vi "调试模式.vi"() -> ()   [LabVIEW 2018]
panel:
  out "开盖指令2":bool
  out "开盖指令1":bool
  out "压紧到位":bool
  out "锁定到位":bool
  out "开盖缓冲":bool
  out "开盖到位2":bool
  out "松开到位":bool
  out "开盖到位1":bool
  out "解锁到位":bool
  out "关盖缓冲":bool
  out "关盖到位2":bool
  out "关盖到位1":bool
  out "关盖指令2":bool
  out "关盖指令1":bool
  out "关盖换向阀":bool
  out "压紧换向阀":bool
  out "松开换向阀":bool
  out "开盖换向阀":bool
  in  "停止":bool
  in  "解锁":bool
  in  "锁定":bool
  in  "压紧":bool
  in  "关盖":bool
  in  "开盖":bool
  in  "松开":bool
  in  "井盖8":bool
  in  "井盖7":bool
  in  "井盖6":bool
  in  "井盖5":bool
  in  "井盖4":bool
  in  "井盖3":bool
  in  "井盖2":bool
  in  "井盖1":bool
  # "显示面板"
  # "操作面板"
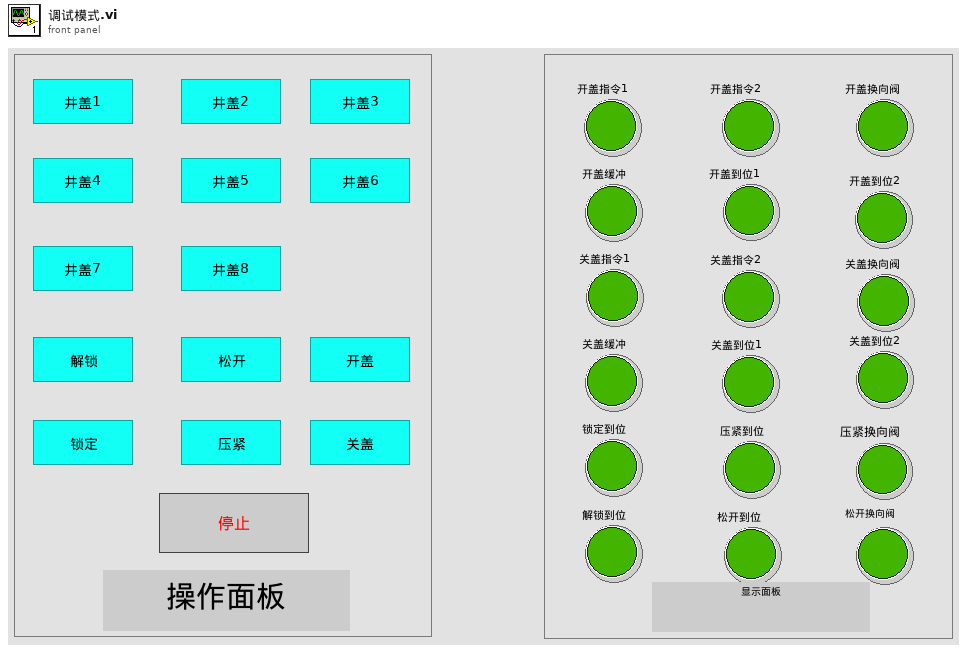
[diagram p1: front panel]
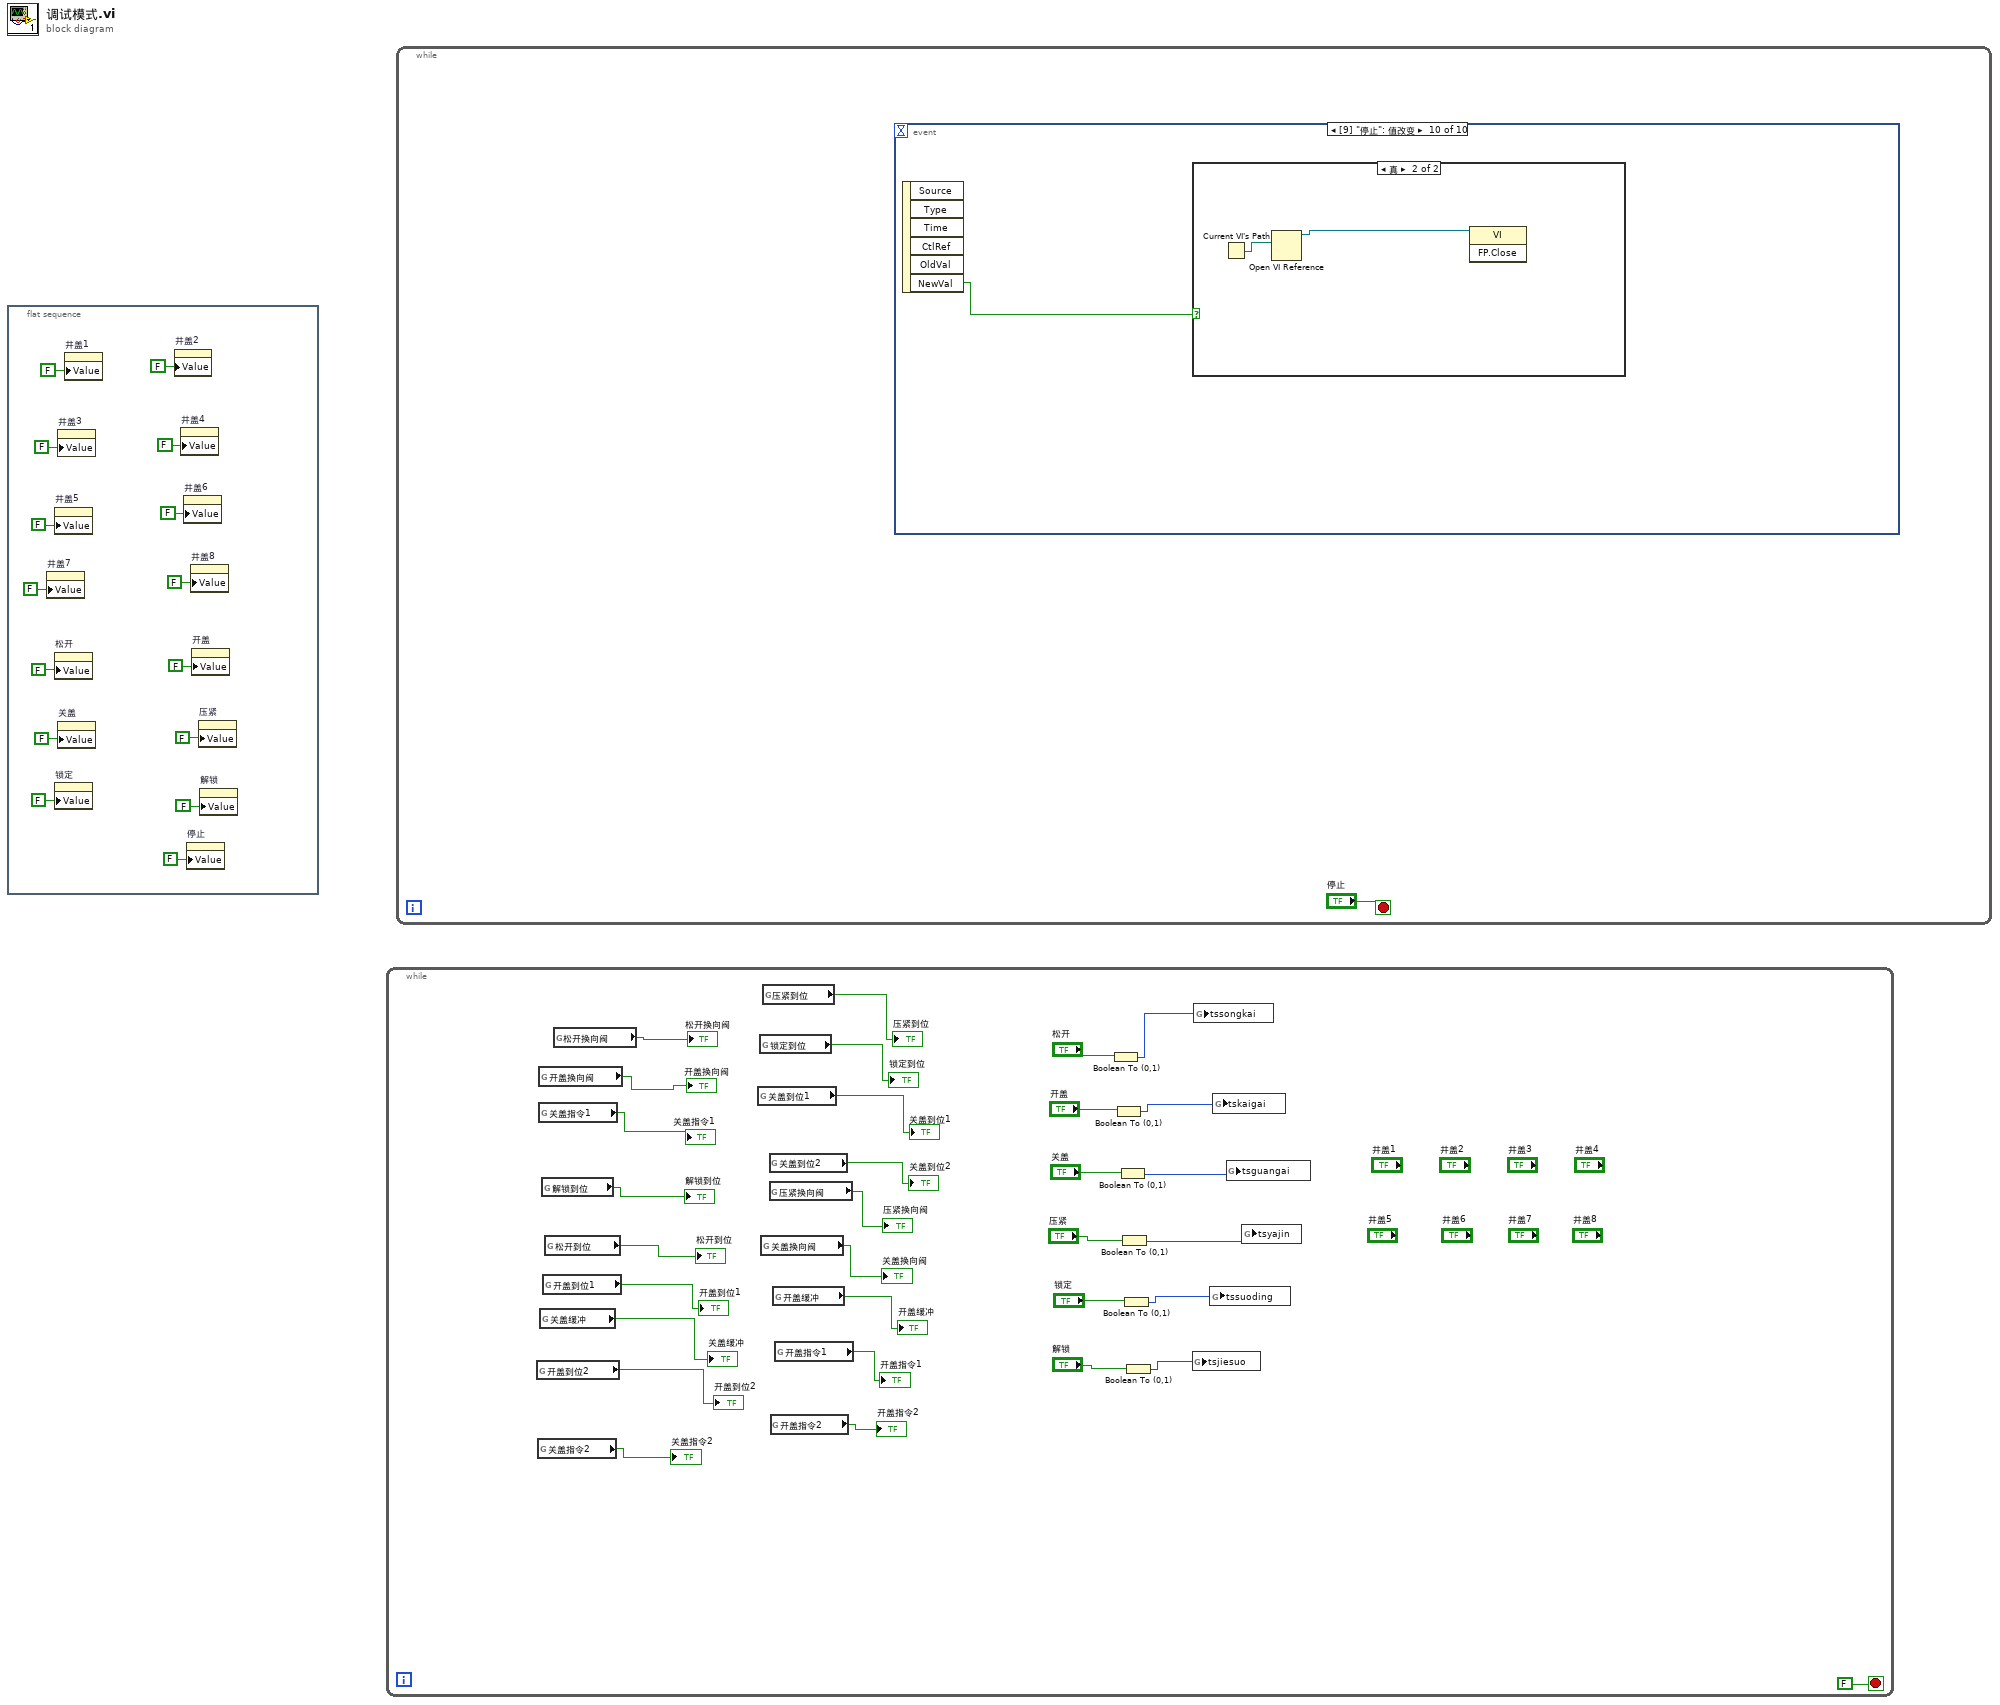
[diagram p0: block diagram]
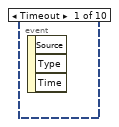
[diagram p2: hidden frame]
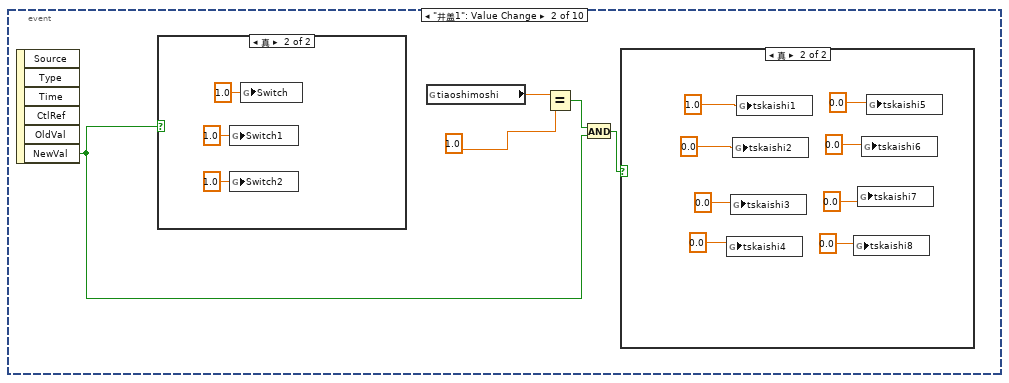
[diagram p3: hidden frame]
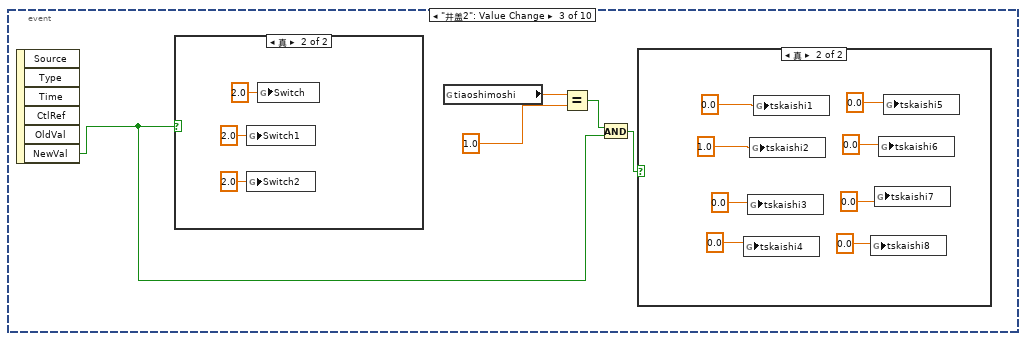
[diagram p6: hidden frame]
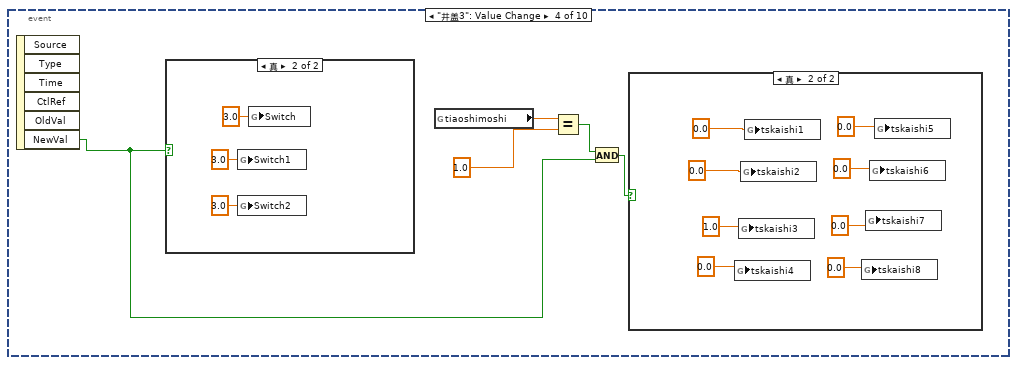
[diagram p9: hidden frame]
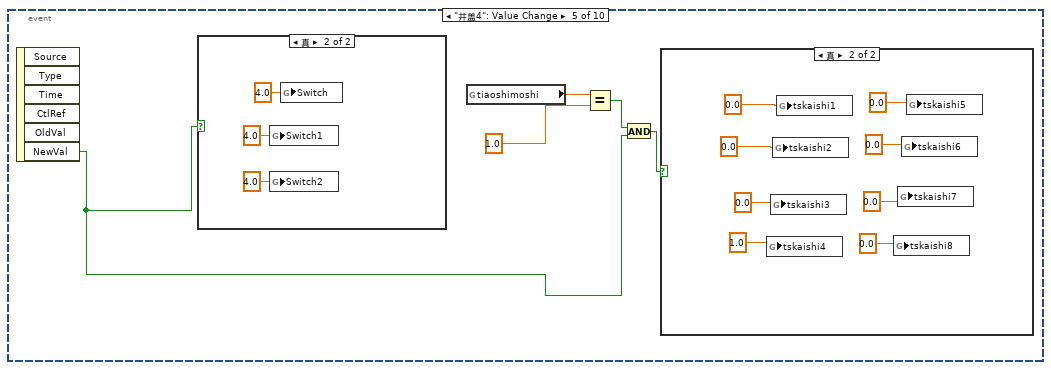
[diagram p12: hidden frame]
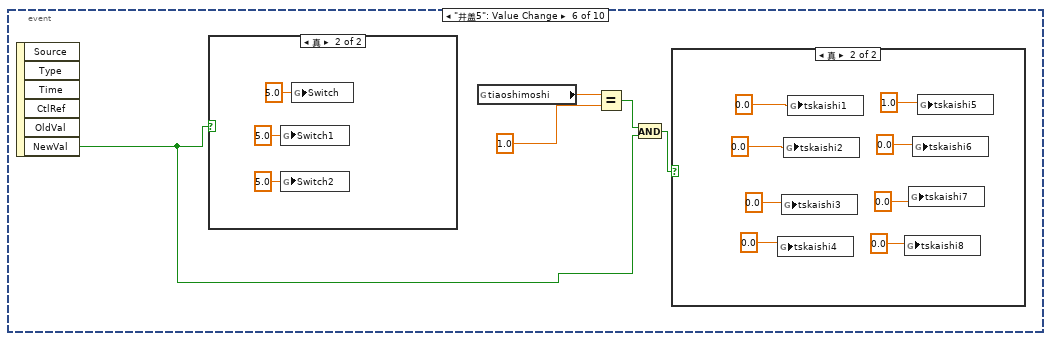
[diagram p15: hidden frame]
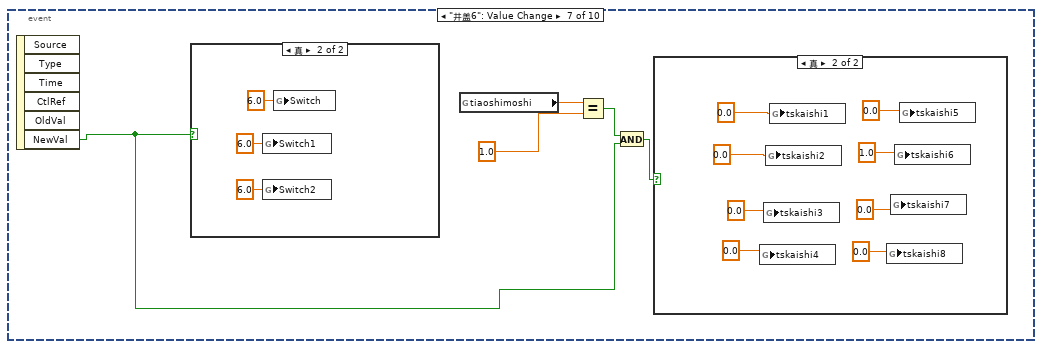
[diagram p18: hidden frame]
diagram:
  n1 = flat-sequence {
    frame #0 {
      n2 = property on="井盖7" class="Bool (严格)"("Value"=FALSE ("井盖7")) -> ()  [unwired: 2 in, 2 out]
      n3 = property on="井盖5" class="Bool (严格)"("Value"=FALSE ("井盖5")) -> ()  [unwired: 2 in, 2 out]
      n4 = property on="松开" class="Bool (严格)"("Value"=FALSE ("松开")) -> ()  [unwired: 2 in, 2 out]
      n5 = property on="锁定" class="Bool (严格)"("Value"=FALSE ("关盖指令")) -> ()  [unwired: 2 in, 2 out]
      n6 = property on="井盖3" class="Bool (严格)"("Value"=FALSE ("井盖3")) -> ()  [unwired: 2 in, 2 out]
      n7 = property on="关盖" class="Bool (严格)"("Value"=FALSE ("关盖")) -> ()  [unwired: 2 in, 2 out]
      n8 = property on="井盖1" class="Bool (严格)"("Value"=FALSE ("井盖1")) -> ()  [unwired: 2 in, 2 out]
      n9 = property on="井盖2" class="Bool (严格)"("Value"=FALSE ("井盖2")) -> ()  [unwired: 2 in, 2 out]
      n10 = property on="井盖4" class="Bool (严格)"("Value"=FALSE ("井盖4")) -> ()  [unwired: 2 in, 2 out]
      n11 = property on="井盖6" class="Bool (严格)"("Value"=FALSE ("井盖6")) -> ()  [unwired: 2 in, 2 out]
      n12 = property on="停止" class="Bool (严格)"("Value"=FALSE ("停止")) -> ()  [unwired: 2 in, 2 out]
      n13 = property on="井盖8" class="Bool (严格)"("Value"=FALSE ("井盖8")) -> ()  [unwired: 2 in, 2 out]
      n14 = property on="开盖" class="Bool (严格)"("Value"=FALSE ("开盖")) -> ()  [unwired: 2 in, 2 out]
      n15 = property on="压紧" class="Bool (严格)"("Value"=FALSE ("压紧")) -> ()  [unwired: 2 in, 2 out]
      n16 = property on="解锁" class="Bool (严格)"("Value"=FALSE ("开盖指令")) -> ()  [unwired: 2 in, 2 out]
    }
  }
  n17 = while {
    stop <- FALSE stop-if-true
    n18 = global read "全局变量.vi" "开盖到位2"() -> (→"开盖到位2":bool)
    n19 = global read "全局变量.vi" "关盖指令2"() -> (→"关盖指令2":bool)
    n20 = global read "全局变量.vi" "开盖换向阀"() -> (→"开盖换向阀":bool)
    n21 = global read "全局变量.vi" "关盖指令1"() -> (→"关盖指令1":bool)
    n22 = global read "全局变量.vi" "关盖缓冲"() -> (→"关盖缓冲":bool)
    n23 = global read "全局变量.vi" "解锁到位"() -> (→"解锁到位":bool)
    n24 = global read "全局变量.vi" "开盖到位1"() -> (→"开盖到位1":bool)
    n25 = global read "全局变量.vi" "松开到位"() -> (→"松开到位":bool)
    n26 = global read "全局变量.vi" "松开换向阀"() -> (→"松开换向阀":bool)
    n27 = global read "全局变量.vi" "关盖到位1"() -> (→"关盖到位1":bool)
    n28 = global read "全局变量.vi" "锁定到位"() -> (→"锁定到位":bool)
    n29 = global read "全局变量.vi" "关盖换向阀"() -> (→"关盖换向阀":bool)
    n30 = global read "全局变量.vi" "压紧到位"() -> (→"压紧到位":bool)
    n31 = global read "全局变量.vi" "关盖到位2"() -> (→"关盖到位2":bool)
    n32 = global read "全局变量.vi" "压紧换向阀"() -> (→"压紧换向阀":bool)
    n33 = global read "全局变量.vi" "开盖指令2"() -> (→"开盖指令2":bool)
    n34 = global read "全局变量.vi" "开盖缓冲"() -> (→"开盖缓冲":bool)
    n35 = global read "全局变量.vi" "开盖指令1"() -> (→"开盖指令1":bool)
    n36 = Boolean To (0,1)(Boolean="松开") -> (0, 1=w22:i16)
    n37 = Boolean To (0,1)(Boolean="开盖") -> (0, 1=w23:i16)
    n38 = Boolean To (0,1)(Boolean="关盖") -> (0, 1=w24:i16)
    n39 = Boolean To (0,1)(Boolean="压紧") -> (0, 1=w25:i16)
    n40 = Boolean To (0,1)(Boolean="锁定") -> (0, 1=w26:i16)
    n41 = Boolean To (0,1)(Boolean="解锁") -> (0, 1=w27:i16)
    n42 = global write "全局变量.vi" "tsjiesuo"(w27) -> ()
    n43 = global write "全局变量.vi" "tssongkai"(w22) -> ()
    n44 = global write "全局变量.vi" "tssuoding"(w26) -> ()
    n45 = global write "全局变量.vi" "tskaigai"(w23) -> ()
    n46 = global write "全局变量.vi" "tsguangai"(w24) -> ()
    n47 = global write "全局变量.vi" "tsyajin"(w25) -> ()
  }
  n48 = while {
    stop <- "停止" stop-if-true
    n49 = event shown="[9] \"停止\": 值改变" {
      selector: _ -> [_ _ _ _ _ _ _ _ _ _]
      dyn-events: _ -> [_ _ _ _ _ _ _ _ _ _]
      timeout: _ -> [_ _ _ _ _ _ _ _ _ _]
      event Timeout {
        n50 = event-data() -> ()  [unwired: 1 in, 3 out]
      }
      event "井盖1": Value Change {
        n51 = event-data() -> ("NewVal"=w49:bool)  [unwired: 1 in, 5 out]
        n52 = case shown="真" w49 {
          frame False {
          }
          frame True {
            n53 = global write "全局变量.vi" "Switch1"(1.0 ("Switch1")) -> ()
            n54 = global write "全局变量.vi" "Switch2"(1.0 ("Switch2")) -> ()
            n55 = global write "全局变量.vi" "Switch"(1.0 ("Switch")) -> ()
          }
        }
        n56 = global read "全局变量.vi" "tiaoshimoshi"() -> (w52:dbl)
        n57 = Equal?(x=w52, y=1.0) -> (x = y?=w50:bool)
        n58 = And(x=w50, y=w49) -> (x .and. y?=w48:bool)
        n59 = case shown="真" w48 {
          frame False {
          }
          frame True {
            n60 = global write "全局变量.vi" "tskaishi4"(0.0 ("Switch")) -> ()
            n61 = global write "全局变量.vi" "tskaishi3"(0.0 ("Switch")) -> ()
            n62 = global write "全局变量.vi" "tskaishi2"(0.0 ("Switch")) -> ()
            n63 = global write "全局变量.vi" "tskaishi1"(1.0 ("Switch")) -> ()
            n64 = global write "全局变量.vi" "tskaishi8"(0.0 ("Switch")) -> ()
            n65 = global write "全局变量.vi" "tskaishi7"(0.0 ("Switch")) -> ()
            n66 = global write "全局变量.vi" "tskaishi6"(0.0 ("Switch")) -> ()
            n67 = global write "全局变量.vi" "tskaishi5"(0.0 ("Switch")) -> ()
          }
        }
      }
      event "井盖2": Value Change {
        n68 = event-data() -> ("NewVal"=w64:bool)  [unwired: 1 in, 5 out]
        n69 = case shown="真" w64 {
          frame False {
          }
          frame True {
            n70 = global write "全局变量.vi" "Switch1"(2.0 ("Switch1")) -> ()
            n71 = global write "全局变量.vi" "Switch2"(2.0 ("Switch2")) -> ()
            n72 = global write "全局变量.vi" "Switch"(2.0 ("Switch")) -> ()
          }
        }
        n73 = global read "全局变量.vi" "tiaoshimoshi"() -> (w68:dbl)
        n74 = Equal?(x=w68, y=1.0) -> (x = y?=w66:bool)
        n75 = And(x=w66, y=w64) -> (x .and. y?=w65:bool)
        n76 = case shown="真" w65 {
          frame False {
          }
          frame True {
            n77 = global write "全局变量.vi" "tskaishi4"(0.0 ("Switch")) -> ()
            n78 = global write "全局变量.vi" "tskaishi3"(0.0 ("Switch")) -> ()
            n79 = global write "全局变量.vi" "tskaishi2"(1.0 ("Switch")) -> ()
            n80 = global write "全局变量.vi" "tskaishi1"(0.0 ("Switch")) -> ()
            n81 = global write "全局变量.vi" "tskaishi8"(0.0 ("Switch")) -> ()
            n82 = global write "全局变量.vi" "tskaishi7"(0.0 ("Switch")) -> ()
            n83 = global write "全局变量.vi" "tskaishi6"(0.0 ("Switch")) -> ()
            n84 = global write "全局变量.vi" "tskaishi5"(0.0 ("Switch")) -> ()
          }
        }
      }
      event "井盖3": Value Change {
        n85 = event-data() -> ("NewVal"=w80:bool)  [unwired: 1 in, 5 out]
        n86 = case shown="真" w80 {
          frame False {
          }
          frame True {
            n87 = global write "全局变量.vi" "Switch1"(3.0 ("Switch1")) -> ()
            n88 = global write "全局变量.vi" "Switch2"(3.0 ("Switch2")) -> ()
            n89 = global write "全局变量.vi" "Switch"(3.0 ("Switch")) -> ()
          }
        }
        n90 = global read "全局变量.vi" "tiaoshimoshi"() -> (w84:dbl)
        n91 = Equal?(x=w84, y=1.0) -> (x = y?=w82:bool)
        n92 = And(x=w82, y=w80) -> (x .and. y?=w81:bool)
        n93 = case shown="真" w81 {
          frame False {
          }
          frame True {
            n94 = global write "全局变量.vi" "tskaishi4"(0.0 ("Switch")) -> ()
            n95 = global write "全局变量.vi" "tskaishi3"(1.0 ("Switch")) -> ()
            n96 = global write "全局变量.vi" "tskaishi2"(0.0 ("Switch")) -> ()
            n97 = global write "全局变量.vi" "tskaishi1"(0.0 ("Switch")) -> ()
            n98 = global write "全局变量.vi" "tskaishi8"(0.0 ("Switch")) -> ()
            n99 = global write "全局变量.vi" "tskaishi7"(0.0 ("Switch")) -> ()
            n100 = global write "全局变量.vi" "tskaishi6"(0.0 ("Switch")) -> ()
            n101 = global write "全局变量.vi" "tskaishi5"(0.0 ("Switch")) -> ()
          }
        }
      }
      event "井盖4": Value Change {
        n102 = event-data() -> ("NewVal"=w96:bool)  [unwired: 1 in, 5 out]
        n103 = case shown="真" w96 {
          frame False {
          }
          frame True {
            n104 = global write "全局变量.vi" "Switch1"(4.0 ("Switch1")) -> ()
            n105 = global write "全局变量.vi" "Switch2"(4.0 ("Switch2")) -> ()
            n106 = global write "全局变量.vi" "Switch"(4.0 ("Switch")) -> ()
          }
        }
        n107 = global read "全局变量.vi" "tiaoshimoshi"() -> (w100:dbl)
        n108 = Equal?(x=w100, y=1.0) -> (x = y?=w98:bool)
        n109 = And(x=w98, y=w96) -> (x .and. y?=w97:bool)
        n110 = case shown="真" w97 {
          frame False {
          }
          frame True {
            n111 = global write "全局变量.vi" "tskaishi4"(1.0 ("Switch")) -> ()
            n112 = global write "全局变量.vi" "tskaishi3"(0.0 ("Switch")) -> ()
            n113 = global write "全局变量.vi" "tskaishi2"(0.0 ("Switch")) -> ()
            n114 = global write "全局变量.vi" "tskaishi1"(0.0 ("Switch")) -> ()
            n115 = global write "全局变量.vi" "tskaishi8"(0.0 ("Switch")) -> ()
            n116 = global write "全局变量.vi" "tskaishi7"(0.0 ("Switch")) -> ()
            n117 = global write "全局变量.vi" "tskaishi6"(0.0 ("Switch")) -> ()
            n118 = global write "全局变量.vi" "tskaishi5"(0.0 ("Switch")) -> ()
          }
        }
      }
      event "井盖5": Value Change {
        n119 = event-data() -> ("NewVal"=w112:bool)  [unwired: 1 in, 5 out]
        n120 = case shown="真" w112 {
          frame False {
          }
          frame True {
            n121 = global write "全局变量.vi" "Switch1"(5.0 ("Switch1")) -> ()
            n122 = global write "全局变量.vi" "Switch2"(5.0 ("Switch2")) -> ()
            n123 = global write "全局变量.vi" "Switch"(5.0 ("Switch")) -> ()
          }
        }
        n124 = global read "全局变量.vi" "tiaoshimoshi"() -> (w116:dbl)
        n125 = Equal?(x=w116, y=1.0) -> (x = y?=w114:bool)
        n126 = And(x=w114, y=w112) -> (x .and. y?=w113:bool)
        n127 = case shown="真" w113 {
          frame False {
          }
          frame True {
            n128 = global write "全局变量.vi" "tskaishi4"(0.0 ("Switch")) -> ()
            n129 = global write "全局变量.vi" "tskaishi3"(0.0 ("Switch")) -> ()
            n130 = global write "全局变量.vi" "tskaishi2"(0.0 ("Switch")) -> ()
            n131 = global write "全局变量.vi" "tskaishi1"(0.0 ("Switch")) -> ()
            n132 = global write "全局变量.vi" "tskaishi8"(0.0 ("Switch")) -> ()
            n133 = global write "全局变量.vi" "tskaishi7"(0.0 ("Switch")) -> ()
            n134 = global write "全局变量.vi" "tskaishi6"(0.0 ("Switch")) -> ()
            n135 = global write "全局变量.vi" "tskaishi5"(1.0 ("Switch")) -> ()
          }
        }
      }
      event "井盖6": Value Change {
        n136 = event-data() -> ("NewVal"=w128:bool)  [unwired: 1 in, 5 out]
        n137 = case shown="真" w128 {
          frame False {
          }
          frame True {
            n138 = global write "全局变量.vi" "Switch1"(6.0 ("Switch1")) -> ()
            n139 = global write "全局变量.vi" "Switch2"(6.0 ("Switch2")) -> ()
            n140 = global write "全局变量.vi" "Switch"(6.0 ("Switch")) -> ()
          }
        }
        n141 = global read "全局变量.vi" "tiaoshimoshi"() -> (w132:dbl)
        n142 = Equal?(x=w132, y=1.0) -> (x = y?=w130:bool)
        n143 = And(x=w130, y=w128) -> (x .and. y?=w129:bool)
        n144 = case shown="真" w129 {
          frame False {
          }
          frame True {
            n145 = global write "全局变量.vi" "tskaishi4"(0.0 ("Switch")) -> ()
            n146 = global write "全局变量.vi" "tskaishi3"(0.0 ("Switch")) -> ()
            n147 = global write "全局变量.vi" "tskaishi2"(0.0 ("Switch")) -> ()
            n148 = global write "全局变量.vi" "tskaishi1"(0.0 ("Switch")) -> ()
            n149 = global write "全局变量.vi" "tskaishi8"(0.0 ("Switch")) -> ()
            n150 = global write "全局变量.vi" "tskaishi7"(0.0 ("Switch")) -> ()
            n151 = global write "全局变量.vi" "tskaishi6"(1.0 ("Switch")) -> ()
            n152 = global write "全局变量.vi" "tskaishi5"(0.0 ("Switch")) -> ()
          }
        }
      }
      event "井盖7": Value Change {
        n153 = event-data() -> ("NewVal"=w144:bool)  [unwired: 1 in, 5 out]
        n154 = case shown="真" w144 {
          frame False {
          }
          frame True {
            n155 = global write "全局变量.vi" "Switch1"(7.0 ("Switch1")) -> ()
            n156 = global write "全局变量.vi" "Switch2"(7.0 ("Switch2")) -> ()
            n157 = global write "全局变量.vi" "Switch"(7.0 ("Switch")) -> ()
          }
        }
        n158 = global read "全局变量.vi" "tiaoshimoshi"() -> (w146:dbl)
        n159 = Equal?(x=w146, y=1.0) -> (x = y?=w147:bool)
        n160 = And(x=w147, y=w144) -> (x .and. y?=w148:bool)
        n161 = case shown="真" w148 {
          frame False {
          }
          frame True {
            n162 = global write "全局变量.vi" "tskaishi4"(0.0 ("Switch")) -> ()
            n163 = global write "全局变量.vi" "tskaishi3"(0.0 ("Switch")) -> ()
            n164 = global write "全局变量.vi" "tskaishi2"(0.0 ("Switch")) -> ()
            n165 = global write "全局变量.vi" "tskaishi1"(0.0 ("Switch")) -> ()
            n166 = global write "全局变量.vi" "tskaishi8"(0.0 ("Switch")) -> ()
            n167 = global write "全局变量.vi" "tskaishi7"(1.0 ("Switch")) -> ()
            n168 = global write "全局变量.vi" "tskaishi6"(0.0 ("Switch")) -> ()
            n169 = global write "全局变量.vi" "tskaishi5"(0.0 ("Switch")) -> ()
          }
        }
      }
      event "井盖8": Value Change {
        n170 = event-data() -> ("NewVal"=w160:bool)  [unwired: 1 in, 5 out]
        n171 = case shown="真" w160 {
          frame False {
          }
          frame True {
            n172 = global write "全局变量.vi" "Switch1"(8.0 ("Switch1")) -> ()
            n173 = global write "全局变量.vi" "Switch2"(8.0 ("Switch2")) -> ()
            n174 = global write "全局变量.vi" "Switch"(8.0 ("Switch")) -> ()
          }
        }
        n175 = global read "全局变量.vi" "tiaoshimoshi"() -> (w164:dbl)
        n176 = Equal?(x=w164, y=1.0) -> (x = y?=w162:bool)
        n177 = And(x=w162, y=w160) -> (x .and. y?=w161:bool)
        n178 = case shown="真" w161 {
          frame False {
          }
          frame True {
            n179 = global write "全局变量.vi" "tskaishi4"(0.0 ("Switch")) -> ()
            n180 = global write "全局变量.vi" "tskaishi3"(0.0 ("Switch")) -> ()
            n181 = global write "全局变量.vi" "tskaishi2"(0.0 ("Switch")) -> ()
            n182 = global write "全局变量.vi" "tskaishi1"(0.0 ("Switch")) -> ()
            n183 = global write "全局变量.vi" "tskaishi8"(1.0 ("Switch")) -> ()
            n184 = global write "全局变量.vi" "tskaishi7"(0.0 ("Switch")) -> ()
            n185 = global write "全局变量.vi" "tskaishi6"(0.0 ("Switch")) -> ()
            n186 = global write "全局变量.vi" "tskaishi5"(0.0 ("Switch")) -> ()
          }
        }
      }
      event "停止": Value Change {
        n187 = event-data() -> ("NewVal"=w176:bool)  [unwired: 1 in, 5 out]
        n188 = case shown="真" w176 {
          frame False {
          }
          frame True {
            n189 = Current VI's Path() -> (path=w178:path)
            n190 = Open VI Reference(vi path=w178) -> (vi reference=w177:refnum<vi>)  [unwired: 5 in, 1 out]
            n191 = invoke class="VI" method="FP.Close"(reference=w177) -> ()  [unwired: 2 in, 3 out]
          }
        }
      }
    }
  }
